vi "Write Window Action Type.vi"(8 "error in (no error)":errorcluster, 10 "Window Action Type":T1, 11 "Window Action in":refnum<class "Window Action.lvclass">) -> (0 "error out":errorcluster, 3 "Window Action out":refnum<class "Window Action.lvclass">)   [LabVIEW 2020, in "MacroAssert.lvlib" / "Window Action.lvclass"]
uses:
  Window Action.lvclass
  Window Action Type.ctl
  Window Action.lvclass/Window Action.ctl
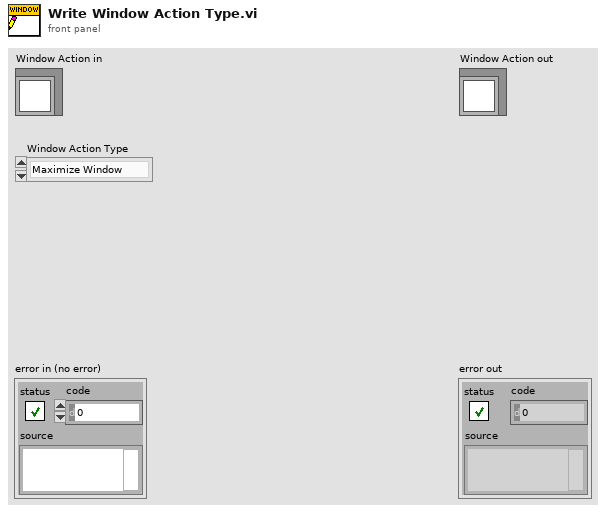
[diagram p1: front panel]
types:
  T1 = typedef "MacroAssert.lvlib/Window Action.lvclass/Window Action Type.ctl" = enum16{"Maximize Window", "Restore Window", "Minimize Window", "Close Window", "Bring Window to Front", "Send Window to Back"}
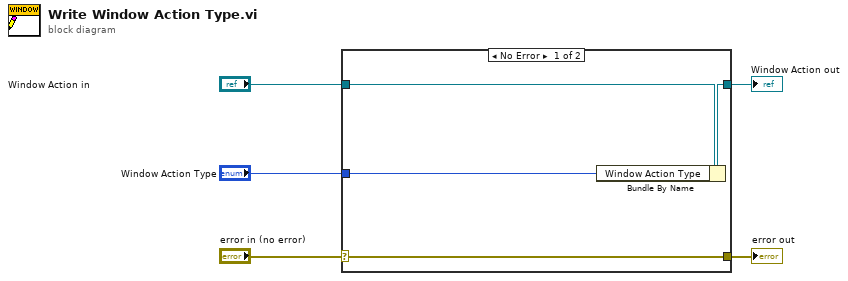
[diagram p0: block diagram]
diagram:
  n1 = case shown="No Error" "error in (no error)" {
    selector: "error in (no error)" -> [w9 w10]
    tunnel: [w9 w10] -> w4
    tunnel: [w7 w11] -> w2
    tunnel: "Window Action in" -> [w8 w11]
    tunnel: "Window Action Type" -> [w6 _]
    frame No Error {
      n2 = Bundle By Name(cluster=w8, "Window Action Type"=w6) -> (w7:refnum<class "Window Action.lvclass">)
    }
    frame Error {
    }
  }
  "error out" <- w4
  "Window Action out" <- w2
